vi "Set Column Order.vi"(8 "error in (no error)":errorcluster, 9 "Destination Column":i32, 10 "Source Column":i32, 11 "UserInterface in":refnum<class "UserInterface.lvclass">) -> (0 "error out":errorcluster, 3 "UserInterface out":refnum<class "UserInterface.lvclass">)   [LabVIEW 2016, in "UserInterface.lvlib" / "UserInterface.lvclass"]
uses:
  UserInterface.lvclass
  UserInterface.lvclass/UserInterface.ctl
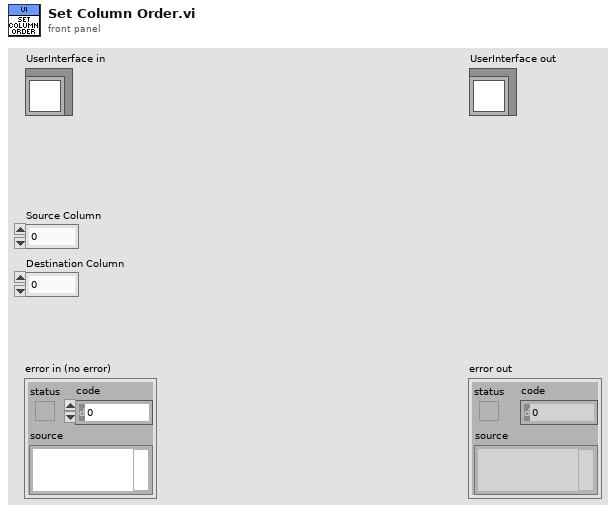
[diagram p1: front panel]
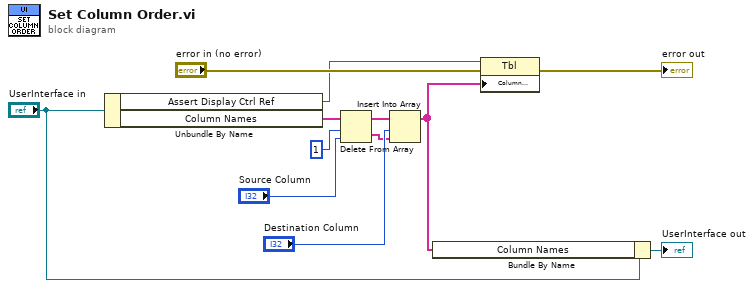
[diagram p0: block diagram]
diagram:
  n1 = Unbundle By Name("UserInterface in") -> ("Assert Display Ctrl Ref"=w4:refnum<vi>, "Column Names"=w8:string[])
  n2 = Delete From Array(array=w8, length=1, index="Source Column") -> (deleted portion=w7:string[], array with subset deleted=w6:string[])
  n3 = Insert Into Array(array=w6, index="Destination Column", new element=w7) -> (w2:string[])
  n4 = Bundle By Name(cluster="UserInterface in", "Column Names"=w2) -> (→"UserInterface out":refnum<class "UserInterface.lvclass">)
  n5 = property class="Tbl"(reference=w4, error in="error in (no error)", "Column Headers[]"=w2) -> (error out=→"error out":errorcluster)  [unwired: 1 out]
